vi "AlliGator Get Array Statistics String.vi"(6 "End String with (\\t)":string="\t", 8 "Error In":errorcluster, 9 "Header Output":bool, 10 "Array Name":string, 11 "Array Statistic":T1) -> (0 "Error Out":errorcluster, 1 "Array Statistics Header String":string, 3 "Array Statistics String":string)   [LabVIEW 2021, in "AlliGator Fit Method Benchmark.lvlib"]
uses:
  AlliGator Fit Method Benchmark.lvlib
  Arrays/Array Statistics.ctl
  Arrays/Arrays.lvlib
panel:
  # "see the License on the block diagram (Ctrl+E or Window:Show Block Diagram)"
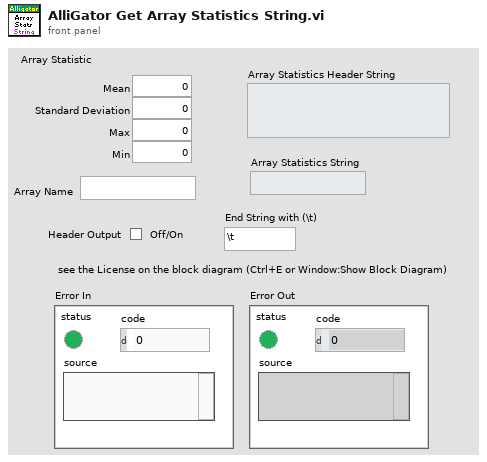
[diagram p1: front panel]
types:
  T1 = typedef "Arrays.lvlib/Array Statistics.ctl" = cluster{"Mean":dbl, "Standard Deviation":dbl, "Max":dbl, "Min":dbl}
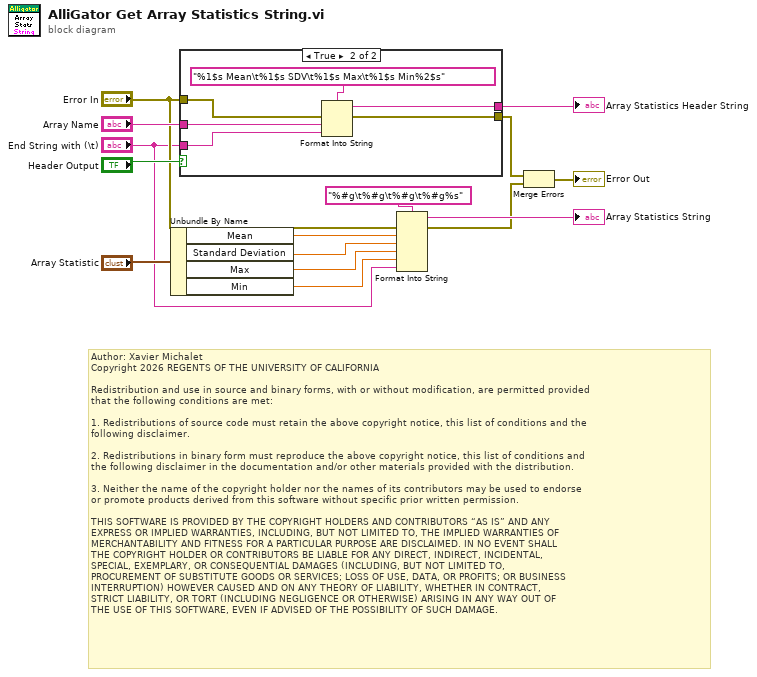
[diagram p0: block diagram]
diagram:
  # "Author: Xavier Michalet\nCopyright 2026 REGENTS OF THE UNIVERSITY OF CALIFORNIA\n\nRedistribution and use in source and binary forms, with or without modification, are permitted provided\nthat the following conditions are met:\n\n1. Redistributions of source code must retain the above copyright notice, this list of conditions and the\nfollowing disclaimer.\n\n2. Redistributions in binary form must reproduce the above copyright notice, this list of conditions and\nthe following disclaimer in the documentation and/or other materials provided with the distribution.\n\n3. Neither the name of the copyright holder nor the names of its contributors may be used to endorse \nor promote products derived from this software without specific prior written permission.\n\nTHIS SOFTWARE IS PROVIDED BY THE COPYRIGHT HOLDERS AND CONTRIBUTORS “AS IS” AND ANY \nEXPRESS OR IMPLIED WARRANTIES, INCLUDING, BUT NOT LIMITED TO, THE IMPLIED WARRANTIES OF\nMERCHANTABILITY AND FITNESS FOR A PARTICULAR PURPOSE ARE DISCLAIMED. IN NO EVENT SHALL\nTHE COPYRIGHT HOLDER OR CONTRIBUTORS BE LIABLE FOR ANY DIRECT, INDIRECT, INCIDENTAL, \nSPECIAL, EXEMPLARY, OR CONSEQUENTIAL DAMAGES (INCLUDING, BUT NOT LIMITED TO, \nPROCUREMENT OF SUBSTITUTE GOODS OR SERVICES; LOSS OF USE, DATA, OR PROFITS; OR BUSINESS\nINTERRUPTION) HOWEVER CAUSED AND ON ANY THEORY OF LIABILITY, WHETHER IN CONTRACT, \nSTRICT LIABILITY, OR TORT (INCLUDING NEGLIGENCE OR OTHERWISE) ARISING IN ANY WAY OUT OF\nTHE USE OF THIS SOFTWARE, EVEN IF ADVISED OF THE POSSIBILITY OF SUCH DAMAGE."
  n1 = Unbundle By Name("Array Statistic") -> ("Mean"=w10:dbl, "Standard Deviation"=w9:dbl, "Max"=w8:dbl, "Min"=w7:dbl)
  n2 = case shown="True" "Header Output" {
    tunnel: "Array Name" -> [_ w21]
    tunnel: "Error In" -> [w16 w20]
    tunnel: [w16 w19] -> w4
    tunnel: [_ w18] -> w12
    tunnel: "End String with (\\t)" -> [_ w17]
    frame False {
    }
    frame True {
      n3 = Format Into String(format string="%1$s Mean\t%1$s SDV\t%1$s Max\t%1$s Min%2$s" ("Array Statistics Header String"), error in=w20, w21, w17) -> (resulting string=w18:string, error out=w19:errorcluster)  [unwired: 1 in]
    }
  }
  "Array Statistics Header String" <- w12
  n4 = Format Into String(format string="%#g\t%#g\t%#g\t%#g%s" ("Array Statistics Header String"), error in="Error In", w10, w9, w8, w7, "End String with (\\t)") -> (resulting string=→"Array Statistics String":string, error out=w3:errorcluster)  [unwired: 1 in]
  n5 = Merge Errors(w4, w3) -> (→"Error Out":errorcluster)
